vi "Set Heater.vi"(6 "Channel":i32, 8 "error in (no error)":errorcluster, 10 "Current (A)":dbl, 11 "Instrument.TC in":refnum<class "Instrument.TC.lvclass">) -> (0 "error out":errorcluster, 3 "Instrument.TC out":refnum<class "Instrument.TC.lvclass">)   [LabVIEW 2019, in "Instrument.TC.lvclass"]
uses:
  Instrument.TC.lvclass
  C:/Program Files (x86)/National Instruments/LabVIEW 2019/user.lib/LevyLab/Instrument Framework/SMOs/Instrument/Instrument.lvclass
  Typedefs/Commands--enum.ctl
  <userlib>/LevyLab/Instrument Framework/Instrument Types/Cryostat/Typedefs/Set Heater--cluster.ctl
  <userlib>/LevyLab/Instrument Framework/SMOs/Instrument/Instrument.lvclass/Instrument.ctl
  6bebe859-88ba-433e-bfb1-01ddf3e256af.vi
  6bebe859-88ba-433e-bfb1-01ddf3e256af.vi/d731064e-7147-48d4-95d8-ab8d0eabd1e4.vi
  <userlib>/LevyLab/Instrument Framework/SMOs/Instrument/API/Send and Receive.vi
  6bebe859-88ba-433e-bfb1-01ddf3e256af.vi/82d3222f-beaa-4f12-aaff-942e256f7958.vi
  <userlib>/LevyLab/Instrument Framework/SMOs/Instrument/Private/Get Client Type.vi
  6bebe859-88ba-433e-bfb1-01ddf3e256af.vi/d731064e-7147-48d4-95d8-ab8d0eabd1e4.vi/be786e68-892b-49ce-8718-6e8a4a025041.vi
  6bebe859-88ba-433e-bfb1-01ddf3e256af.vi/d731064e-7147-48d4-95d8-ab8d0eabd1e4.vi/ad4dbca0-acb5-4f86-98c4-89ee27f16455.vi
  6bebe859-88ba-433e-bfb1-01ddf3e256af.vi/82d3222f-beaa-4f12-aaff-942e256f7958.vi/1b65f6bd-5912-49c2-98e1-d9ee56444d91.vi
  6bebe859-88ba-433e-bfb1-01ddf3e256af.vi/82d3222f-beaa-4f12-aaff-942e256f7958.vi/e1d8c442-0bc2-404e-8346-12030aacea5b.vi
  6bebe859-88ba-433e-bfb1-01ddf3e256af.vi/82d3222f-beaa-4f12-aaff-942e256f7958.vi/1b65f6bd-5912-49c2-98e1-d9ee56444d91.vi/47d72b3f-ba1b-4795-b6a2-602052193040.vi
  6bebe859-88ba-433e-bfb1-01ddf3e256af.vi/82d3222f-beaa-4f12-aaff-942e256f7958.vi/1b65f6bd-5912-49c2-98e1-d9ee56444d91.vi/d8a2b507-1651-49df-b443-3f0ea086789f.vi
  <userlib>/LevyLab/Instrument Framework/SMOs/Instrument/Private/Get RC Connection Status.vi
  <userlib>/LevyLab/Instrument Framework/SMOs/Instrument/API/Enum to String.vi
  <userlib>/LevyLab/Instrument Framework/SMOs/RemoteControl/API/Send and Receive.vi
  <vilib>/Utility/Data Type/Get Type Information.vi
  <vilib>/JDP Science/JSONtext/JSON text to Variant.vi
  <userlib>/LevyLab/Instrument Framework/SMOs/Instrument/API/Instrument.GetPublicEvents.vi
  <vilib>/JDP Science/JSONtext/Variant to JSON Text.vi
  <vilib>/National Instruments/GUID Generator/Guid Generator.vi
  <userlib>/LevyLab/Instrument Framework/SMOs/Instrument/API/Instrument.MessageToProcess.vi
  <userlib>/LevyLab/Instrument Framework/SMOs/Instrument/Private/Instrument.MessageFromProcess.EventStructure.vi
  <vilib>/JDP Science/JSONtext/LVClass Serializer/JSONtext LVClass Serializer.lvclass
  <userlib>/LevyLab/Instrument Framework/Instrument Types/Cryostat/Instrument.Cryostat.lvclass
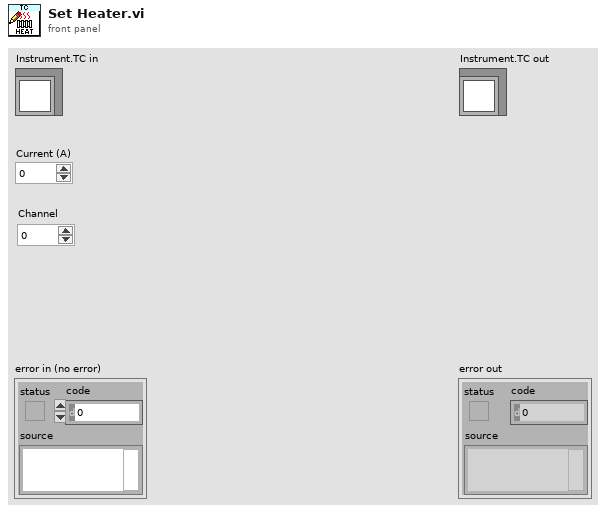
[diagram p1: front panel]
types:
  T1 = typedef "Instrument.Cryostat.lvclass/Set Heater--cluster.ctl" = cluster{"Channel":i32, "Current (A)":dbl}
  T2 = typedef "Instrument.TC.lvclass/Commands--enum.ctl" = enum16{"Set Heater"}
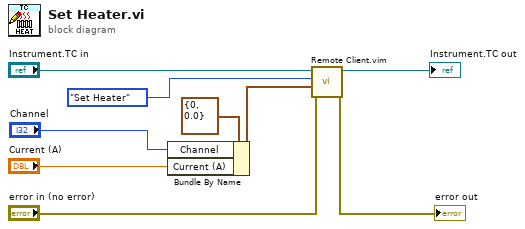
[diagram p0: block diagram]
diagram:
  n1 = Bundle By Name(cluster=T1 {"Channel"=0, "Current (A)"=0.0} ("Set Heater"), "Channel"="Channel", "Current (A)"="Current (A)") -> (w1:T1)
  n2 = call "Remote Client.vim"("error in (no error)"="error in (no error)", "params"=w1, "method"=Commands--enum."Set Heater" ("Commands"), "Instrument in"="Instrument.TC in") -> ("error out"=→"error out":errorcluster, "Instrument out"=→"Instrument.TC out":refnum<class "Instrument.TC.lvclass">)  [unwired: 4 in, 2 out]
